vi "Sign Test.vi"   [LabVIEW 2020, in "NI_Gmath.lvlib"]
doc: "Tests hypotheses about the <B>median</B> of continuous distributions. You must manually select the polymorphic instance to use."
uses:
  NI_Gmath.lvlib
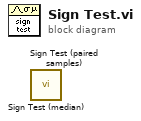
[diagram p0: block diagram]
diagram:
  n1 = call "Sign Test (median).vi"() -> ()  [unwired: 9 in, 3 out]
  n2 = call "Sign Test (paired samples).vi"() -> ()  [unwired: 9 in, 3 out]
